vi "Create Host String.vi"(6 "URL formatting":T1=enum."region.", 7 "Include Default Region":bool, 8 "Redirect Endpoint":string, 9 "URL Prefix":string, 10 "Region":string, 11 "AWS Service":string) -> (3 "Host String":string)   [LabVIEW 2015, in "NI_AWS_Core.lvlib" / "HTTP Request.lvclass"]
uses:
  HTTP Request.lvclass
  URL formatting.ctl
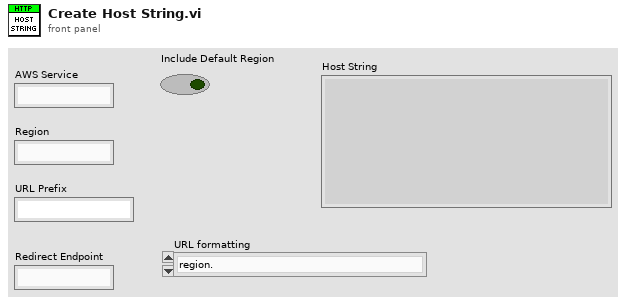
[diagram p1: front panel]
types:
  T1 = typedef "NI_AWS_Core.lvlib/HTTP Request.lvclass/URL formatting.ctl" = enum16{"region-", "region."}
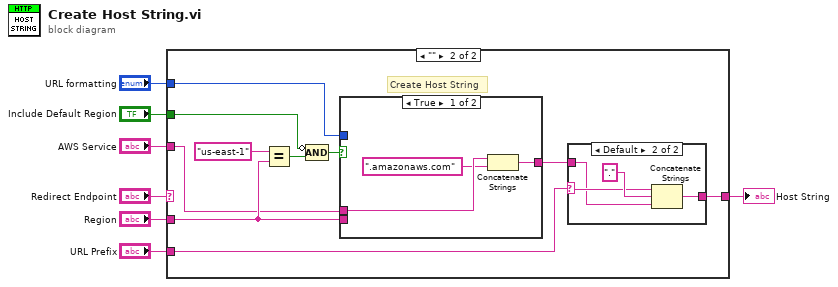
[diagram p0: block diagram]
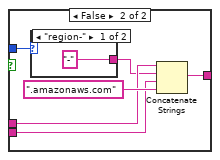
[diagram p3: hidden frame]
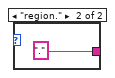
[diagram p4: hidden frame]
diagram:
  n1 = case shown="\"\"" "Redirect Endpoint" {
    selector: "Redirect Endpoint" -> [w8 _]
    tunnel: [w8 w14] -> w7
    tunnel: "AWS Service" -> [_ w10]
    tunnel: "Region" -> [_ w13]
    tunnel: "URL Prefix" -> [_ w12]
    tunnel: "URL formatting" -> [_ w11]
    tunnel: "Include Default Region" -> [_ w9]
    frame Default {
    }
    frame "" {
      # "Create Host String"
      n2 = Equal?(x="us-east-1", y=w13) -> (x = y?=w15:bool)
      n3 = Compound Arithmetic op=AND(invert w9, w15) -> (w17:bool)
      n4 = case shown="True" w17 {
        tunnel: [w21 w27] -> w18
        tunnel: w10 -> [w20 w24]
        tunnel: w13 -> [_ w25]
        tunnel: w11 -> [_ w23]
        frame True {
          n5 = Concatenate Strings(w20, ".amazonaws.com" ("string")) -> (w21:string)
        }
        frame False {
          n6 = case shown="\"region-\"" w23 {
            tunnel: ["-" ("string") "." ("string")] -> w22
            frame "region-" {
            }
            frame "region." {
            }
          }
          n7 = Concatenate Strings(w24, w22, w25, ".amazonaws.com" ("string")) -> (w27:string)
        }
      }
      n8 = case shown="Default" w12 {
        selector: w12 -> [_ w32]
        tunnel: [w30 w34] -> w14
        tunnel: w18 -> [w30 w31]
        frame "" {
        }
        frame Default {
          n9 = Concatenate Strings(w32, "." ("string"), w31) -> (w34:string)
        }
      }
    }
  }
  "Host String" <- w7
